vi "LVFunction_LoadFilePMC.vi"() -> ()   [LabVIEW 2020]
panel:
  in  "PathToWavefrontCorrectorSetupFile":path
  out "error out":errorcluster
  in  "error in (no error)":errorcluster
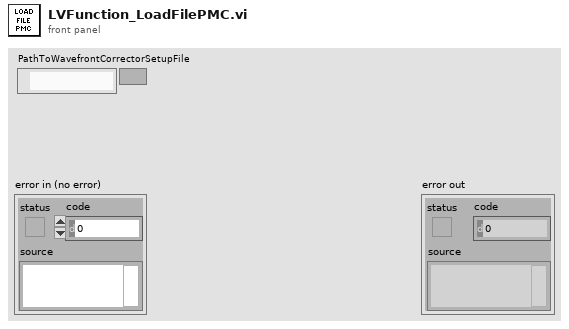
[diagram p1: front panel]
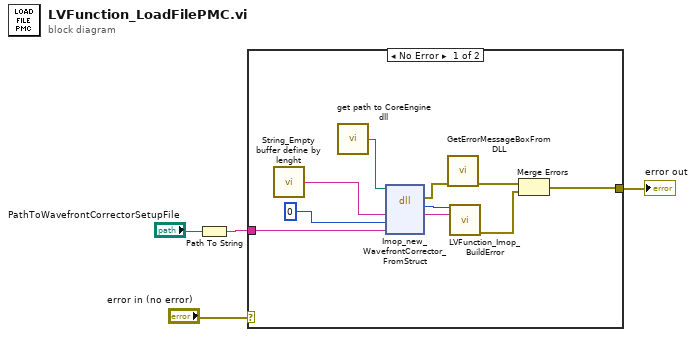
[diagram p0: block diagram]
diagram:
  n1 = Path To String(path="PathToWavefrontCorrectorSetupFile") -> (string=w4:string)
  n2 = case shown="No Error" "error in (no error)" {
    selector: "error in (no error)" -> [_ w15]
    tunnel: [w13 w15] -> w2
    tunnel: w4 -> [w14 _]
    frame No Error {
      n3 = call "String_Empty buffer define by lenght.vi"() -> ("Empty buffer"=w12:string)  [unwired: 1 in]
      n4 = call "get path to CoreEngine dll.vi"() -> ("path to c_interface_vc100.dll"=w9:path)  [unwired: 12 in, 3 out]
      n5 = dll-call lib="D:/soft/HASO_v3/C_interface/Sources/Build/vc100/Release/c_interface_vc100.dll" fn="Imop_new_WavefrontCorrector_FromStruct"(path in=w9, "message"=w12, "WavefrontCorrector"=0 ("Pupil"), "Config_file_path"=w14) -> (error out=w8:errorcluster, "return type"=w10:i32, "message"=w11:string)  [unwired: 4 in, 1 out]
      n6 = call "GetErrorMessageBoxFromDLL.vi"("error IN"=w8) -> ("error OUT"=w6:errorcluster)  [unwired: 10 in]
      n7 = call "LVFunction_Imop_BuildError.vi"("code"=w10, "String to Prepend to source (\"\")"=w11) -> ("error out"=w5:errorcluster)  [unwired: 13 in]
      n8 = Merge Errors(w6, w5) -> (w13:errorcluster)
    }
    frame Error {
    }
  }
  "error out" <- w2
